vi "IsMatch.vi"(8 "error in (no error)":errorcluster, 9 "Item to match":refnum<class "ILabVIEWItem.lvclass">, 11 "CItemMatch in":refnum<class "CItemMatch.lvclass">) -> (0 "error out":errorcluster, 1 "Is match?":bool, 3 "CItemMatch out":refnum<class "CItemMatch.lvclass">)   [LabVIEW 2020, in "DependencyInspection.lvlib" / "CItemMatch.lvclass"]
uses:
  CItemMatch.lvclass
  obj/Addons/LabVIEWObjectInterfaces.lvlibp/LabVIEWObjectInterfaces/ILabVIEWItem/ILabVIEWItem.lvclass
  CItemMatch.lvclass/CItemMatch.ctl
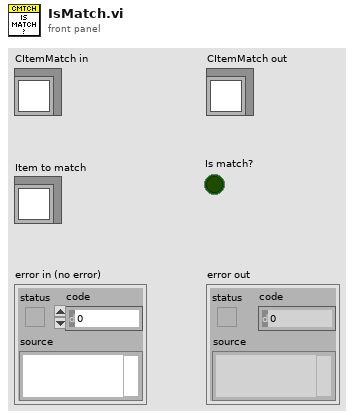
[diagram p1: front panel]
types:
  T1 = typedef "DependencyInspection.lvlib/CItemMatch.lvclass/Field.ctl" = enum16{"Name", "Qualified name", "Path"}
  T2 = typedef "DependencyInspection.lvlib/CItemMatch.lvclass/ComparisonType.ctl" = enum16{"None", "Ends with", "Equals", "Not equal", "Starts with", "Contains", "Matches pattern"}
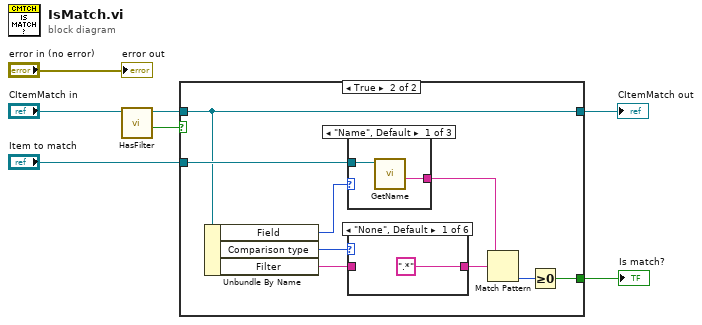
[diagram p0: block diagram]
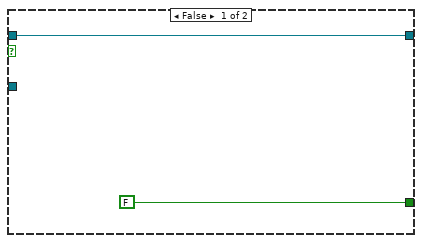
[diagram p2: hidden frame]
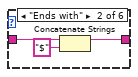
[diagram p3: hidden frame]
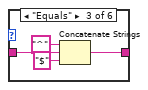
[diagram p4: hidden frame]
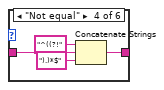
[diagram p5: hidden frame]
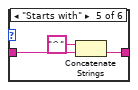
[diagram p6: hidden frame]
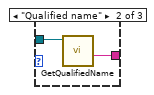
[diagram p8: hidden frame]
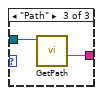
[diagram p9: hidden frame]
diagram:
  n1 = call-dynamic "HasFilter.vi"("CItemMatch in"="CItemMatch in") -> ("Has filter?"=w1:bool, "CItemMatch out"=w3:refnum<class "CItemMatch.lvclass">)  [unwired: 8 in, 1 out]
  n2 = case shown="True" w1 {
    tunnel: "Item to match" -> [_ w18]
    tunnel: [FALSE w14] -> w5
    tunnel: w3 -> [w8 w10]
    tunnel: [w8 w10] -> w2
    frame False {
    }
    frame True {
      n3 = Unbundle By Name(w10) -> ("Field"=w13:T1, "Comparison type"=w12:T2, "Filter"=w11:string)
      n4 = case shown="\"Name\", Default" w13 {
        tunnel: w18 -> [w36 w38 w40]
        tunnel: [w35 w37 w39] -> w17
        frame "Name", Default {
          n5 = call-dynamic "GetName.vi"("ILabVIEWItem in"=w36) -> ("Name"=w35:string)  [unwired: 8 in, 2 out]
        }
        frame "Qualified name" {
          n6 = call-dynamic "GetQualifiedName.vi"("ILabVIEWItem in"=w38) -> ("Qualified name"=w37:string)  [unwired: 8 in, 2 out]
        }
        frame "Path" {
          n7 = call-dynamic "GetPath.vi"("ILabVIEWItem in"=w40) -> ("Path"=w39:string)  [unwired: 8 in, 2 out]
        }
      }
      n8 = case shown="\"None\", Default" w12 {
        tunnel: w11 -> [_ w22 w26 w30 w33 w34]
        tunnel: [".*" w20 w24 w28 w32 w34] -> w16
        frame "None", Default {
        }
        frame "Ends with" {
          n9 = Concatenate Strings(w22, "$" ("string")) -> (w20:string)
        }
        frame "Equals" {
          n10 = Concatenate Strings("^" ("string"), w26, "$" ("string")) -> (w24:string)
        }
        frame "Not equal" {
          n11 = Concatenate Strings("^((?!" ("string"), w30, ").)*$" ("string")) -> (w28:string)
        }
        frame "Starts with" {
          n12 = Concatenate Strings("^" ("string"), w33) -> (w32:string)
        }
        frame "Contains", "Matches pattern" {
        }
      }
      n13 = Match Pattern(string=w17, regular expression=w16) -> (offset past match=w15:i32)  [unwired: 1 in, 3 out]
      n14 = Greater Or Equal To 0?(x=w15) -> (x >= 0?=w14:bool)
    }
  }
  "CItemMatch out" <- w2
  "Is match?" <- w5
  "error out" <- "error in (no error)"
